vi "Get 1D I64.vi"(7 "key description":string, 8 "sections":string[](array[string]), 9 "numeric":i64[](array[numeric]), 11 "info data":string) -> (0 "sections out":string[](array[string]), 1 "key found?":bool, 2 "value":i64[](array[numeric]), 3 "info data out":string)   [LabVIEW 2020, in "infolib.lvlib"]
doc: "Add a new numeric key to Info Data string. If section exists in Info Data string, inserts key into this section."
uses:
  infolib.lvlib
  Get 2D I64.vi
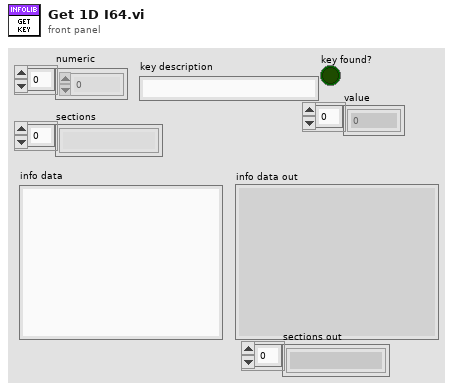
[diagram p1: front panel]
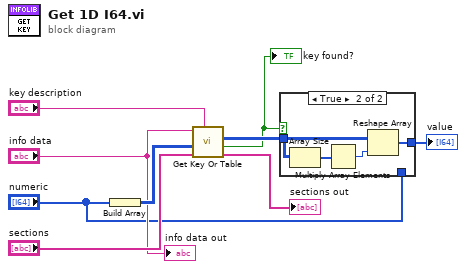
[diagram p0: block diagram]
diagram:
  n1 = Build Array("numeric") -> (w8:i64[][])
  n2 = call-poly "Get Key Or Table.vi"("key description"="key description", "sections"="sections", "numeric"=w8, "info data"="info data") -> ("sections out"=→"sections out":string[], "key found?"=w2:bool, "value"=w4:i64[][])  [unwired: 4 in, 1 out]
  "key found?" <- w2
  n3 = case shown="True" w2 {
    tunnel: w4 -> [_ w12]
    tunnel: [w10 w11] -> w3
    tunnel: "numeric" -> [w10 _]
    frame False {
    }
    frame True {
      n4 = Array Size(array=w12) -> (size(s)=w13:i32[])
      n5 = Multiply Array Elements(1:w13) -> (0:w14:i32)
      n6 = Reshape Array(w12, w14) -> (w11:i64[])
    }
  }
  "value" <- w3
  "info data out" <- "info data"
